vi "teleop.vi"(10 "Match Info":T1={"Autonomous Elapsed Seconds"=0.0, "TeleOp Elapsed Seconds"=0.0, "Disabled Elapsed Seconds"=0.0, "Visited Autonomous"=FALSE, "Visited TeleOp"=FALSE, "Visited Disabled"=FALSE, "Autonomous Settings"={"Autonomous Style"=enum."Independent", "VI Refnum"=refnum}}, 11 "Call Context":T2) -> ()   [LabVIEW 2012]
doc: "This VI is called for each TeleOp packet received from the DS where the robot is not disabled. It is often used to read from the joysticks and update I/O or to update setpoints for timed control loops. It should complete and return within 20 milliseconds or it may miss DS packets."
uses:
  <vilib>/Rock Robotics/WPI/DriverStation/WPI_DriverStationDerivedRobotMode.ctl
  <vilib>/Rock Robotics/WPI/DriverStation/WPI_DriverStationMatch Info.ctl
  Robot Global Data.vi
  System Set Points and States.vi
  <vilib>/Rock Robotics/WPI/Joystick/WPI_JoystickGetSetRefNum.vi
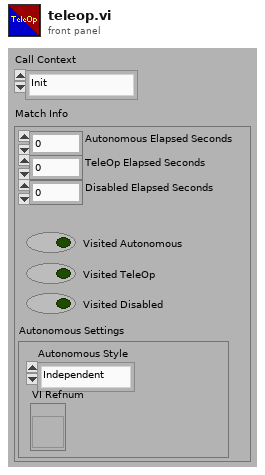
[diagram p1: front panel]
types:
  T1 = typedef "WPI_DriverStationMatch Info.ctl" = cluster{"Autonomous Elapsed Seconds":dbl, "TeleOp Elapsed Seconds":dbl, "Disabled Elapsed Seconds":dbl, "Visited Autonomous":bool, "Visited TeleOp":bool, "Visited Disabled":bool, "Autonomous Settings":cluster{"Autonomous Style":enum16{"Iterative", "Independent"}, "VI Refnum":refnum<vi>}}
  T2 = typedef "WPI_DriverStationDerivedRobotMode.ctl" = enum16{"Init", "Execute", "Stop"}
  T3 = typedef "WPI_JoystickDevRef.ctl" = cluster{"Device":T4}
  T4 = typedef "WPI_JoystickDeviceEnum.ctl" = enum16{"USB 1", "USB 2", "USB 3", "USB 4", "Kinect 1", "Kinect 2"}
  T5 = typedef "WPI_JoystickButtonState.ctl" = cluster{"Button 1":bool, "Button 2":bool, "Button 3":bool, "Button 4":bool, "Button 5":bool, "Button 6":bool, "Button 7":bool, "Button 8":bool, "Button 9":bool, "Button 10":bool, "Button 11":bool, "Button 12":bool}
  T6 = cluster{"axis 1 (x)":dbl, "axis 2 (y)":dbl, "axis 3 (throttle)":dbl, "axis 4":dbl, "axis 5":dbl, "axis 6":dbl}
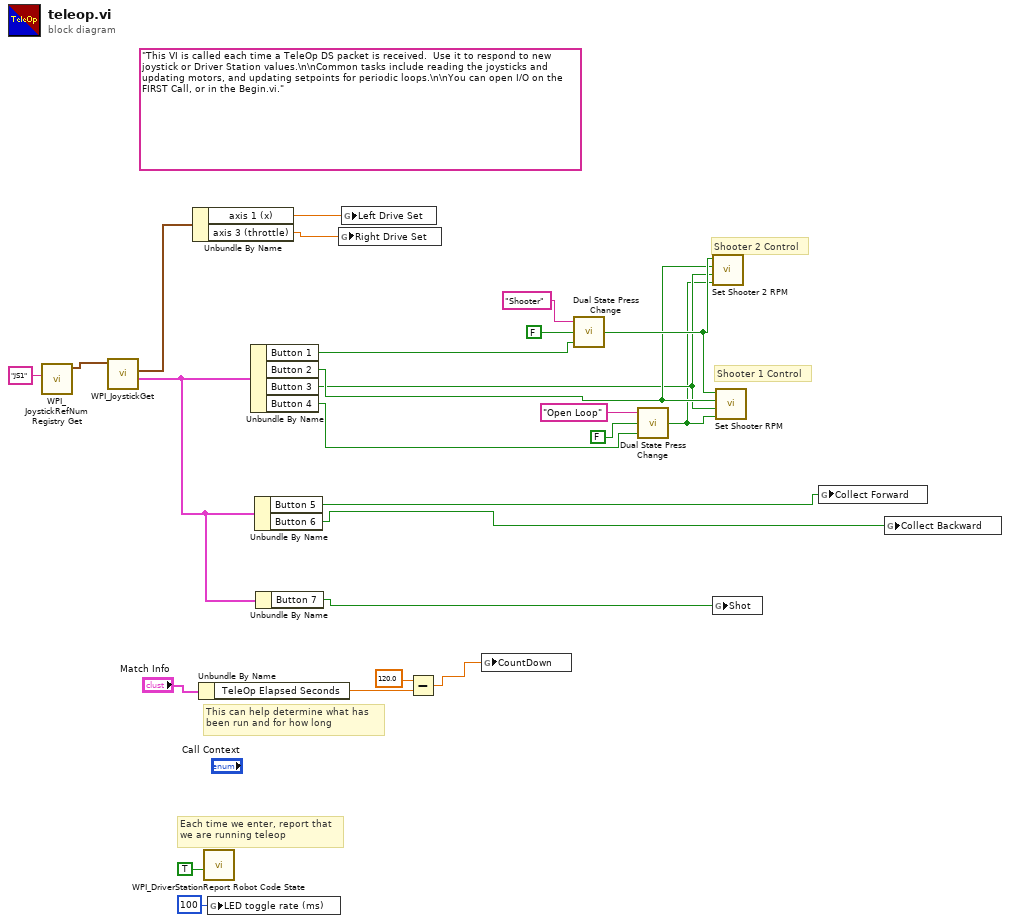
[diagram p0: block diagram]
diagram:
  (unwired) "This VI is called each time a TeleOp DS packet is received.  Use it to respond to new joystick or Driver Station values.\n\nCommon tasks include reading the joysticks and updating motors, and updating setpoints for periodic loops.\n\nYou can open I/O on the FIRST Call, or in the Begin.vi."
  # "Shooter 2 Control"
  # "Shooter 1 Control"
  # "Each time we enter, report that\nwe are running teleop"
  # "This can help determine what has\nbeen run and for how long"
  n1 = call <vilib>:"WPI_JoystickRefNum Registry Get.vi"("refnum name"="JS1") -> ("JoystickDevRef"=w15:T3)  [unwired: 9 in, 1 out]
  n2 = call <vilib>:"WPI_JoystickGet.vi"("JoystickDevRef"=w15) -> ("Buttons"=w4:T5, "Axes"=w14:T6)  [unwired: 4 in, 1 out]
  n3 = Unbundle By Name(w14) -> ("axis 1 (x)"=w2:dbl, "axis 3 (throttle)"=w1:dbl)
  n4 = Unbundle By Name("Match Info") -> ("TeleOp Elapsed Seconds"=w19:dbl)
  n5 = call <vilib>:"WPI_DriverStationReport Robot Code State.vi"("TeleOp"=TRUE ("Autonomous")) -> ()  [unwired: 10 in, 1 out]
  n6 = global write "Robot Global Data.vi" "LED toggle rate (ms)"(u32 100 ("LED ms toggle rate")) -> ()
  n7 = Unbundle By Name(w4) -> ("Button 1"=w12:bool, "Button 2"=w9:bool, "Button 3"=w8:bool, "Button 4"=w11:bool)
  n8 = Unbundle By Name(w4) -> ("Button 5"=w6:bool, "Button 6"=w5:bool)
  n9 = Unbundle By Name(w4) -> ("Button 7"=w3:bool)
  n10 = global write "System Set Points and States.vi" "Right Drive Set"(w1) -> ()
  n11 = global write "System Set Points and States.vi" "Left Drive Set"(w2) -> ()
  n12 = Subtract(x=120.0, y=w19) -> (x-y=w17:dbl)
  n13 = global write "System Set Points and States.vi" "CountDown"(w17) -> ()
  n14 = call "Dual State Press Change.vi"("Enable/Disable"=w12, "Initial"=FALSE, "Value Name"="Shooter") -> ("Enabled"=w10:bool)
  n15 = call "Dual State Press Change.vi"("Enable/Disable"=w11, "Initial"=FALSE, "Value Name"="Open Loop") -> ("Enabled"=w7:bool)
  n16 = call "Set Shooter 2 RPM.vi"("Open Loop"=w7, "Increment"=w8, "Decrement"=w9, "Shooter Enabled"=w10) -> ()  [unwired: 8 in]
  n17 = global write "System Set Points and States.vi" "Shot"(w3) -> ()
  n18 = call "Set Shooter RPM.vi"("Open Loop"=w7, "Increment"=w8, "Decrement"=w9, "Shooter Enabled"=w10) -> ()  [unwired: 8 in]
  n19 = global write "System Set Points and States.vi" "Collect Forward"(w6) -> ()
  n20 = global write "System Set Points and States.vi" "Collect Backward"(w5) -> ()
